vi "lookupService.vi"(5 "Service ROS":T2={"topic port"=0, "Node"="", "topic"="", "type"="", "node port"=0, "error "={"status"=FALSE, "code"=0, "source"=""}, "Direction"=enum."Node", "APIs"=[], "Update (ms)"=1, "write queue"=1}) -> (0 "error out":errorcluster, 1 "Log":T1)   [LabVIEW 2012]
uses:
  _ROSDefinition.vi
  Console/Servers/ServerSubs/MyState.ctl
  Console/Servers/ServerSubs/ROSLog.ctl
  SubVIs/_ROSDirection.ctl
  SubVIs/_ROSControl.ctl
panel:
  out "response":string
  out "lookupService":string="POST /RPC2 HTTP/1.1\r\nHost: 192.168.1.110:11311\r\nContent-Type: text/xml\r\nContent-Length: 396\r\n\r\n<?xml version='1.0'?>\n<methodCall>\r <methodName>registerSubscriber</methodName>\r <params>\r   <param><value><string>/ChrisAir</string> </value> </param>\r   <param><value><string>/robot/joint_states</string> </value> </param>\r   <param><value><string>sensor_msgs/JointState</string> </value> </param>\r   <param><value><string>http://192.168.1.111</string> </value> </param>\r </params>\r</methodCall>"
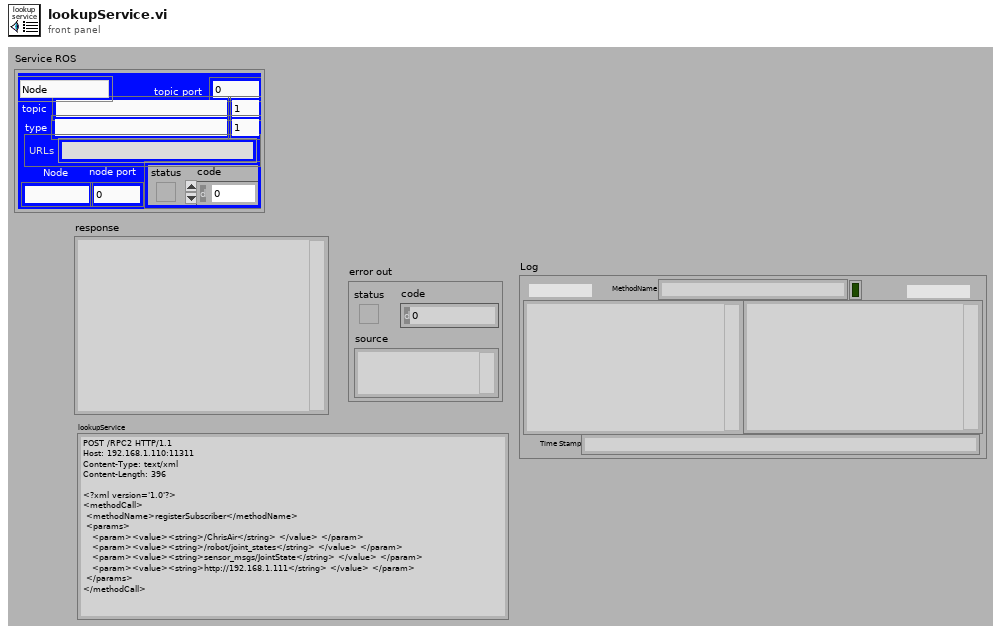
[diagram p1: front panel]
types:
  T1 = typedef "ROSLog.ctl" = cluster{"Sent":string, "Reply":string, "MethodName":string, "success":bool, "Dir1":string, "Dir2":string, "Time Stamp":string}
  T2 = typedef "_ROSControl.ctl" = cluster{"topic port":u16, "Node":string, "topic":string, "type":string, "node port":u32, "error ":errorcluster, "Direction":T3, "APIs":string[], "Update (ms)":u16, "write queue":u16}
  T3 = typedef "_ROSDirection.ctl" = enum16{"Node", "Publisher", "Subscriber", "Service Client"}
  T4 = typedef "MyState.ctl" = enum16{"No Connection", "Registered", "Connected", "Close"}
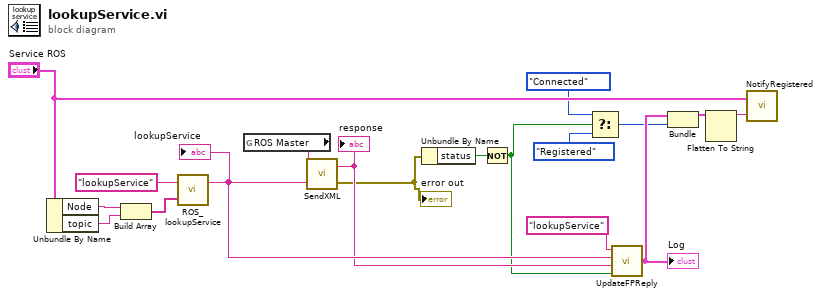
[diagram p0: block diagram]
diagram:
  n1 = Unbundle By Name("Service ROS") -> ("Node"=w18:string, "topic"=w17:string)
  n2 = Build Array(w18, w17) -> (w16:string[])
  n3 = call "ROS_lookupService.vi"("Parameters"=w16, "Method Name"="lookupService") -> ("lookupService"=w14:string)  [unwired: 1 in]
  "lookupService" <- w14
  n4 = global read "_ROSDefinition.vi" "ROS Master"() -> (w10:string)
  n5 = call "SendXML.vi"("Send"=w14, "URI in"=w10) -> ("error out"=w7:errorcluster, "Reply"=w13:string)
  "error out" <- w7
  "response" <- w13
  n6 = Unbundle By Name(w7) -> ("status"=w11:bool)
  n7 = Not(x=w11) -> (.not. x?=w4:bool)
  n8 = Select(t=MyState."Connected" ("MyState"), s=w4, f=MyState."Registered" ("MyState")) -> (s? t:f=w1:T4)
  n9 = call "UpdateFPReply.vi"("success?"=w4, "Reply"=w13, "Sent"=w14, "method"="lookupService" ("Method Name")) -> ("Log"=w6:T1)
  "Log" <- w6
  n10 = Bundle("Log"=w6, "MyState"=w1) -> (w5:cluster{"Log":T1, "MyState":T4})  [unwired: 1 in]
  n11 = Flatten To String(anything=w5) -> (data string=w9:string)  [unwired: 3 in, 2 out]
  n12 = call "NotifyRegistered.vi"("data string"=w9, "ROS"="Service ROS") -> ()  [unwired: 2 in]
